vi "SWERVE_MODULE_ACT.vi"(4 "Steering Vel FF Kn":dbl=1.0 format="%#_13g", 5 "Drive Motor Info":T2={"Motor Name"="LF Drive", "MC type"=enum."Talon FX, P5", "Motor Type"=enum."NEO", "Gear Ratio"=0.0}, 6 "Drive Vel FF Kn":dbl=1.0 format="%#_13g", 7 "Steering Motor Info":T2={"Motor Name"="LF Steering", "MC type"=enum."Talon FX, P5", "Motor Type"=enum."NEO", "Gear Ratio"=0.0}, 8 "dt_Sec":dbl=0.02 format="%#_13g", 9 "Wheel Diameter IN":dbl=4.0 format="%#_13g", 10 "Swerve State":T3={"Speed"=0.0, "Angle"={"VALUE"=0.0, "COS"=1.0, "SIN"=0.0}} {"Angle"."SIN" format="%13.4f"; "Angle"."COS" format="%13.4f"; "Angle"."VALUE" format="%13.4f"}, 11 "Swerve Dmd":T3={"Speed"=0.0, "Angle"={"VALUE"=0.0, "COS"=1.0, "SIN"=0.0}} {"Angle"."SIN" format="%13.4f"; "Angle"."COS" format="%13.4f"; "Angle"."VALUE" format="%13.4f"}) -> ()   [LabVIEW 2023]
doc: "Creates a new SwerveModuleAct for an individual module with the specified swerve module state demand. \n\nParameters\n - Drive Vel FF Kn -- The normalization constant for Velocity FF on the Drive Motor.\n - Steering Vel FF Kn -- The normalization constant for Velocity FF on the Steering Motor."
uses:
  <vilib>/Rock Robotics/WPI/ThirdParty/JAS_Junk/TrajLib/TypeDef/SWERVE_DRIVE_MODULE_STATE.ctl
  <vilib>/Rock Robotics/WPI/ThirdParty/JAS_Junk/TrajLib/TypeDef/ROTATION2D.ctl
  <vilib>/Rock Robotics/WPI/ThirdParty/JAS_Junk/TrajLib/Enum/DCMOTOR_TYPES_ENUM.ctl
  <vilib>/Rock Robotics/WPI/ThirdParty/JAS_Junk/TrajLib/TypeDef/DCMOTOR_SIM.ctl
  <vilib>/Rock Robotics/WPI/ThirdParty/JAS_Junk/TrajLib/TypeDef/LINEAR_SYSTEM_SIM.ctl
  <vilib>/Rock Robotics/WPI/ThirdParty/JAS_Junk/TrajLib/TypeDef/LINEAR_SYSTEM.ctl
  <vilib>/Analysis/Matrix/Datatypes/RealMatrix.ctl
  <vilib>/Rock Robotics/WPI/ThirdParty/JAS_Junk/TrajLib/TypeDef/DCMOTOR.CTL
  <vilib>/Rock Robotics/WPI/ThirdParty/JAS_Junk/TrajLib/MathUtil_InputModulus.vi
  <vilib>/Rock Robotics/WPI/ThirdParty/JAS_Junk/TrajLib/DCMotor_GetCIM.vi
  <vilib>/Rock Robotics/WPI/ThirdParty/JAS_Junk/TrajLib/DCMotor_GetAndymark9015.vi
  <vilib>/Rock Robotics/WPI/ThirdParty/JAS_Junk/TrajLib/DCMotor_GetAndymarkRs775_125.vi
  <vilib>/Rock Robotics/WPI/ThirdParty/JAS_Junk/TrajLib/DCMotor_GetBag.vi
  <vilib>/Rock Robotics/WPI/ThirdParty/JAS_Junk/TrajLib/DCMotor_GetBanebotsRs550.vi
  <vilib>/Rock Robotics/WPI/ThirdParty/JAS_Junk/TrajLib/DCMotor_GetBanebotsRs775.vi
  <vilib>/Rock Robotics/WPI/ThirdParty/JAS_Junk/TrajLib/DCMotor_GetFalcon500.vi
  <vilib>/Rock Robotics/WPI/ThirdParty/JAS_Junk/TrajLib/DCMotor_GetMiniCIM.vi
  <vilib>/Rock Robotics/WPI/ThirdParty/JAS_Junk/TrajLib/DCMotor_GetNEO.vi
  <vilib>/Rock Robotics/WPI/ThirdParty/JAS_Junk/TrajLib/DCMotor_GetNEO550.vi
  <vilib>/Rock Robotics/WPI/ThirdParty/JAS_Junk/TrajLib/DCMotor_GetRomiBuiltIn.vi
  <vilib>/Rock Robotics/WPI/ThirdParty/JAS_Junk/TrajLib/DCMotor_GetVex775Pro.vi
  <vilib>/Rock Robotics/WPI/ThirdParty/JAS_Junk/TrajLib/VI/DCMotor_GetAndymarkAM2235A.vi
  <vilib>/Rock Robotics/WPI/ThirdParty/JAS_Junk/TrajLib/VI/DCMotor_GetAndymarkAM3493.vi
  <vilib>/Rock Robotics/WPI/ThirdParty/JAS_Junk/TrajLib/VI/DCMotor_GetFalcon500_FOC.vi
  <vilib>/Rock Robotics/WPI/ThirdParty/JAS_Junk/TrajLib/VI/DCMotor_GetKrakenX60.vi
  <vilib>/Rock Robotics/WPI/ThirdParty/JAS_Junk/TrajLib/VI/DCMotor_GetKrakenX60_FOC.vi
  <vilib>/Rock Robotics/WPI/ThirdParty/JAS_Junk/TrajLib/VI/DCMotor_GetNEOVortex.vi
  <vilib>/Rock Robotics/WPI/ThirdParty/JAS_Junk/TrajLib/Conv_Inches_Meters.vi
  <vilib>/Rock Robotics/WPI/ThirdParty/JAS_Junk/TrajLib/ProfiledPIDController_SetPID.vi
  <vilib>/Rock Robotics/WPI/ThirdParty/JAS_Junk/TrajLib/ProfiledPIDController_SetIntegratorRange.vi
  <vilib>/Rock Robotics/WPI/ThirdParty/JAS_Junk/TrajLib/ProfiledPIDController_SetTolerance_PosVel.vi
  <vilib>/Rock Robotics/WPI/ThirdParty/JAS_Junk/TrajLib/ProfiledPIDController_DisableContInput.vi
  <vilib>/Rock Robotics/WPI/ThirdParty/JAS_Junk/TrajLib/ProfiledPIDController_EnableContInput.vi
  <vilib>/Rock Robotics/WPI/ThirdParty/JAS_Junk/TrajLib/ProfiledPIDController_Reset_PosOnly.vi
  <vilib>/Rock Robotics/WPI/ThirdParty/JAS_Junk/TrajLib/ProfiledPIDController_NewPeriod.vi
  <vilib>/Rock Robotics/WPI/ThirdParty/JAS_Junk/TrajLib/ProfiledPIDController_Calculate_Meas_Goal.vi
  <vilib>/Rock Robotics/WPI/ThirdParty/JAS_Junk/TrajLib/ProfiledPIDController_AtGoal.vi
  <vilib>/Rock Robotics/WPI/ThirdParty/JAS_Junk/TrajLib/ProfiledPIDController_AtSetpoint.vi
  <vilib>/Rock Robotics/WPI/ThirdParty/JAS_Junk/TrajLib/ProfiledPIDController_SetConstraints.vi
  <vilib>/Rock Robotics/WPI/ThirdParty/JAS_Junk/TrajLib/SimpleMotorFF_Calculate.vi
  <vilib>/Rock Robotics/WPI/ThirdParty/JAS_Junk/TrajLib/PIDController_AtSetpoint.vi
  <vilib>/Rock Robotics/WPI/ThirdParty/JAS_Junk/TrajLib/PIDController_SetPIDF.vi
  <vilib>/Rock Robotics/WPI/ThirdParty/JAS_Junk/TrajLib/PIDController_SetDerivativeFilter.vi
  <vilib>/Rock Robotics/WPI/ThirdParty/JAS_Junk/TrajLib/PIDController_SetIntegratorRange.vi
  <vilib>/Rock Robotics/WPI/ThirdParty/JAS_Junk/TrajLib/PIDController_SetTolerancePandV.vi
  <vilib>/Rock Robotics/WPI/ThirdParty/JAS_Junk/TrajLib/PIDController_DisableContinousInput.vi
  <vilib>/Rock Robotics/WPI/ThirdParty/JAS_Junk/TrajLib/PIDController_EnableContinousInput.vi
  <vilib>/Rock Robotics/WPI/ThirdParty/JAS_Junk/TrajLib/PIDController_Reset.vi
  <vilib>/Rock Robotics/WPI/ThirdParty/JAS_Junk/TrajLib/PIDController_New.vi
  <vilib>/Rock Robotics/WPI/ThirdParty/JAS_Junk/TrajLib/PIDController_SetOutputLimits.vi
  <vilib>/Rock Robotics/WPI/ThirdParty/JAS_Junk/TrajLib/VI/PIDController_SetIntegratorZone.vi
  <vilib>/Rock Robotics/WPI/ThirdParty/JAS_Junk/TrajLib/DCMotor_New.vi
  <vilib>/Rock Robotics/WPI/ThirdParty/JAS_Junk/TrajLib/PIDController_SetPID.vi
  <vilib>/Rock Robotics/WPI/ThirdParty/JAS_Junk/TrajLib/TrapProfState_New.vi
  <vilib>/Rock Robotics/WPI/ThirdParty/JAS_Junk/TrajLib/ProfiledPIDController_Reset.vi
  <vilib>/Rock Robotics/WPI/ThirdParty/JAS_Junk/TrajLib/PIDController_NewPeriod.vi
  <vilib>/Rock Robotics/SystemInterfaces/NetworkCommunication/NetComm_UsageReport_report.vi
  <vilib>/Rock Robotics/WPI/ThirdParty/JAS_Junk/TrajLib/ProfiledPIDController_SetGoal_PosOnly.vi
  <vilib>/Rock Robotics/WPI/ThirdParty/JAS_Junk/TrajLib/ProfiledPIDController_Calculate_Meas.vi
  <vilib>/Rock Robotics/WPI/ThirdParty/JAS_Junk/TrajLib/TrapProfState_Equals.vi
  <vilib>/Rock Robotics/WPI/ThirdParty/JAS_Junk/TrajLib/ProfiledPIDController_SetGoal.vi
  <vilib>/Rock Robotics/WPI/ThirdParty/JAS_Junk/TrajLib/PIDController_Calculate_SP_PV.vi
  <vilib>/Rock Robotics/WPI/ThirdParty/JAS_Junk/TrajLib/TrapProfile_New.vi
  <vilib>/Rock Robotics/WPI/ThirdParty/JAS_Junk/TrajLib/ProfiledPIDController_GetPeriod.vi
  <vilib>/Rock Robotics/WPI/ThirdParty/JAS_Junk/TrajLib/TrapProfile_Calculate.vi
  <vilib>/Rock Robotics/WPI/ThirdParty/JAS_Junk/TrajLib/ControllerUtil_GetModulusError.vi
  <vilib>/Rock Robotics/WPI/ThirdParty/JAS_Junk/TrajLib/PIDController_SetSetpoint.vi
  <vilib>/Rock Robotics/WPI/ThirdParty/JAS_Junk/TrajLib/PIDController_Calculate_PV.vi
  <vilib>/Rock Robotics/WPI/ThirdParty/JAS_Junk/TrajLib/TrapProfile_ShouldFlipAcceleration.vi
  <vilib>/Rock Robotics/WPI/ThirdParty/JAS_Junk/TrajLib/TrapProfile_Direct.vi
  <vilib>/Rock Robotics/WPI/ThirdParty/JAS_Junk/TrajLib/PIDController_GetPeriod.vi
  <vilib>/Rock Robotics/Network Tables/NT Read Variant.vi
  <vilib>/Rock Robotics/WPI/ThirdParty/JAS_Junk/TrajLib/Globals/Util_LibraryGlobals.vi
  <vilib>/Rock Robotics/Network Tables/NT Write Variant.vi
  <vilib>/Rock Robotics/WPI/ThirdParty/JAS_Junk/TrajLib/PIDController_AdvCalculate_FF_Sp_Pv.vi
  <vilib>/Rock Robotics/WPI/ThirdParty/Phoenix-LabVIEW/Motor Controller/Controls/CTRE_Phoenix_MotorControl_ControlMode.ctl
  <vilib>/Rock Robotics/WPI/ThirdParty/JAS_Junk/TrajLib/Trajectory_Library.lvlib
  <vilib>/Rock Robotics/WPI/ThirdParty/REV Robotics/REVLib/Typedef/Spark MAX Control Type.ctl
  <vilib>/Analysis/Matrix/NI_Matrix.lvlib
  <vilib>/Rock Robotics/WPI/ThirdParty/Phoenix6/controls/VelocityDutyCycle SetControl.vi
  <vilib>/Rock Robotics/WPI/ThirdParty/Phoenix6/getters/GetPRO_PosAndVel_Position.vi
  <vilib>/Rock Robotics/WPI/ThirdParty/Phoenix6/controls/PositionDutyCycle SetControl.vi
  <vilib>/Rock Robotics/WPI/ThirdParty/Phoenix6/getters/GetPRO_PosAndVel_Velocity.vi
  <vilib>/Rock Robotics/WPI/ThirdParty/Phoenix-LabVIEW/Motor Controller/Get/CTRE_Phoenix_MotorController_GetSelectedSensorData.vi
  <vilib>/Rock Robotics/WPI/ThirdParty/REV Robotics/REVLib/SubVI/Public/SPARK Get Encoder Status Position.vi
  <vilib>/Rock Robotics/WPI/ThirdParty/REV Robotics/REVLib/SubVI/Public/SPARK Get Encoder Status Velocity.vi
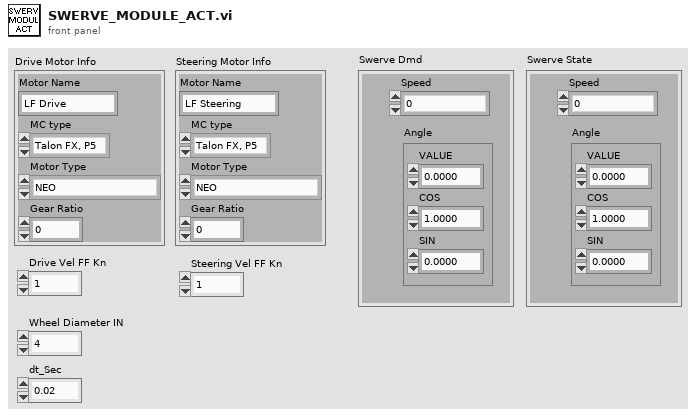
[diagram p1: front panel]
types:
  T1 = typedef "Trajectory_Library.lvlib/DCMOTOR_TYPES_ENUM.ctl" = enum16{"CIM", "AndyMark 9015", "Andy Mark RS 775 125", "Bag", "BaneBots RS 550", "BaneBots RS 775", "Falcon 500", "Mini CIM", "NEO", "NEO 550", "Romi BuiltIn", "Vex 775 Pro", "Snow Blower AM 2235A", "Bosch Seat AM 3493", "Falcon 500 FOC", "Kraken X60", "Kraken X60 FOC", "NEO Vortex"}
  T2 = cluster{"Motor Name":string, "MC type":enum16{"Talon FX, P5", "Talon FX, P6", "SPARK MAX"}, "Motor Type":T1, "Gear Ratio":dbl}
  T3 = typedef "Trajectory_Library.lvlib/SWERVE_DRIVE_MODULE_STATE.ctl" = cluster{"Speed":dbl, "Angle":T4}
  T4 = typedef "Trajectory_Library.lvlib/ROTATION2D.ctl" = cluster{"VALUE":dbl, "COS":dbl, "SIN":dbl}
  T5 = enum16{"Talon FX, P5", "Talon FX, P6", "SPARK MAX"}
  T6 = enum16{"DemandType_Neutral", "DemandType_AuxPID", "DemandType_ArbitraryFeedForward"}
  T7 = typedef "Spark MAX Control Type.ctl" = enum16{"Percent VBus", "Voltage", "Velocity", "Position", "Smart Motion", "Current", "Smart Velocity", "MAXMotion Position", "MAXMotion Velocity"}
  T8 = cluster{"Future Proof Configs":bool, "MotorOutputInverted":u16, "MotorOutputNeutralMode":u16, "MotorOutputDutyCycleNeutralDeadband":dbl, "MotorOutputPeakForwardDutyCycle":dbl, "MotorOutputPeakReverseDutyCycle":dbl, "MotorOutputControlTimesyncFreqHz":dbl, "CurrentLimitsStatorCurrentLimit":dbl, "CurrentLimitsStatorCurrentLimitEnable":bool, "CurrentLimitsSupplyCurrentLimit":dbl, "CurrentLimitsSupplyCurrentLimitEnable":bool, "CurrentLimitsSupplyCurrentLowerLimit":dbl, "CurrentLimitsSupplyCurrentLowerTime":dbl, "VoltageSupplyVoltageTimeConstant":dbl, "VoltagePeakForwardVoltage":dbl, "VoltagePeakReverseVoltage":dbl, "TorqueCurrentPeakForwardTorqueCurrent":dbl, "TorqueCurrentPeakReverseTorqueCurrent":dbl, "TorqueCurrentTorqueNeutralDeadband":dbl, "FeedbackFeedbackRotorOffset":dbl, "FeedbackSensorToMechanismRatio":dbl, "FeedbackRotorToSensorRatio":dbl, "FeedbackFeedbackSensorSource":u16, "FeedbackFeedbackRemoteSensorID":i16, "FeedbackVelocityFilterTimeConstant":dbl, "DifferentialSensorsDifferentialSensorSource":u16, "DifferentialSensorsDifferentialTalonFXSensorID":i16, "DifferentialSensorsDifferentialRemoteSensorID":i16, "DifferentialConstantsPeakDifferentialDutyCycle":dbl, "DifferentialConstantsPeakDifferentialVoltage":dbl, "DifferentialConstantsPeakDifferentialTorqueCurrent":dbl, "OpenLoopRampsDutyCycleOpenLoopRampPeriod":dbl, "OpenLoopRampsVoltageOpenLoopRampPeriod":dbl, "OpenLoopRampsTorqueOpenLoopRampPeriod":dbl, "ClosedLoopRampsDutyCycleClosedLoopRampPeriod":dbl, "ClosedLoopRampsVoltageClosedLoopRampPeriod":dbl, "ClosedLoopRampsTorqueClosedLoopRampPeriod":dbl, "HardwareLimitSwitchForwardLimitType":u16, "HardwareLimitSwitchForwardLimitAutosetPositionEnable":bool, "HardwareLimitSwitchForwardLimitAutosetPositionValue":dbl, "HardwareLimitSwitchForwardLimitEnable":bool, "HardwareLimitSwitchForwardLimitSource":u16, "HardwareLimitSwitchForwardLimitRemoteSensorID":i16, "HardwareLimitSwitchReverseLimitType":u16, "HardwareLimitSwitchReverseLimitAutosetPositionEnable":bool, "HardwareLimitSwitchReverseLimitAutosetPositionValue":dbl, "HardwareLimitSwitchReverseLimitEnable":bool, "HardwareLimitSwitchReverseLimitSource":u16, "HardwareLimitSwitchReverseLimitRemoteSensorID":i16, "AudioBeepOnBoot":bool, "AudioBeepOnConfig":bool, "AudioAllowMusicDurDisable":bool, "SoftwareLimitSwitchForwardSoftLimitEnable":bool, "SoftwareLimitSwitchReverseSoftLimitEnable":bool, "SoftwareLimitSwitchForwardSoftLimitThreshold":dbl, "SoftwareLimitSwitchReverseSoftLimitThreshold":dbl, "MotionMagicMotionMagicCruiseVelocity":dbl, "MotionMagicMotionMagicAcceleration":dbl, "MotionMagicMotionMagicJerk":dbl, "MotionMagicMotionMagicExpo_kV":dbl, "MotionMagicMotionMagicExpo_kA":dbl, "CustomParamsCustomParam0":i16, "CustomParamsCustomParam1":i16, "ClosedLoopGeneralContinuousWrap":bool, "Slot0kP":dbl, "Slot0kI":dbl, "Slot0kD":dbl, "Slot0kS":dbl, "Slot0kV":dbl, "Slot0kA":dbl, "Slot0kG":dbl, "Slot0GravityType":u16, "Slot0StaticFeedforwardSign":u16, "Slot1kP":dbl, "Slot1kI":dbl, "Slot1kD":dbl, "Slot1kS":dbl, "Slot1kV":dbl, "Slot1kA":dbl, "Slot1kG":dbl, "Slot1GravityType":u16, "Slot1StaticFeedforwardSign":u16, "Slot2kP":dbl, "Slot2kI":dbl, "Slot2kD":dbl, "Slot2kS":dbl, "Slot2kV":dbl, "Slot2kA":dbl, "Slot2kG":dbl, "Slot2GravityType":u16, "Slot2StaticFeedforwardSign":u16}
  T9 = typedef "Trajectory_Library.lvlib/DCMOTOR_SIM.ctl" = cluster{"LinearSystemSim":T10, "GearBox":T13, "Gearing":dbl}
  T10 = typedef "Trajectory_Library.lvlib/LINEAR_SYSTEM_SIM.ctl" = cluster{"m_Plant":T11, "m_X":T12, "m_Y":T12, "m_U":T12, "MeasureStdDev":T12}
  T11 = typedef "Trajectory_Library.lvlib/LINEAR_SYSTEM.ctl" = cluster{"m_A":T12, "m_B":T12, "m_C":T12, "m_D":T12, "States":i32, "Inputs":i32, "Outputs":i32}
  T12 = typedef "NI_Matrix.lvlib/RealMatrix.ctl" = dbl[][]
  T13 = typedef "Trajectory_Library.lvlib/DCMOTOR.CTL" = cluster{"nominalVoltage_Volts":dbl, "StallTorque_NM":dbl, "StallCurrent_Amps":dbl, "FreeCurrent_Amps":dbl, "FreeSpeed_RadPerSec":dbl, "R_Ohms":dbl, "KvINV_RadPerSecPerVolt":dbl, "Kt_NMPerAmp":dbl, "L_H":dbl, "Jr_KgM2":dbl}
  T14 = typedef "CTRE_Phoenix_MotorControl_ControlMode.ctl" = u16
  T15 = typedef "Trajectory_Library.lvlib/SIMPLE_MOTOR_FF.ctl" = cluster{"Ks":dbl, "Kv":dbl, "Ka":dbl, "KnInv":dbl}
  T16 = typedef "WPI_MotorControlDeviceRef.ctl" = cluster{"DeviceStatus":errorcluster, "Type":T17, "PWM":cluster{"PWM Channel":T18, "DeadBand":T19}, "CAN":cluster{"Device Number":u8, "SetOutput VI Ref":variant, "GetOutput VI Ref":variant, "Enable VI Ref":variant, "Disable VI Ref":variant, "Data":variant}, "Invert":bool, "DIO PWM":cluster{"PWM \"Enable\" Channel":T18, "DIOChannel":T20, "PWM Rate":dbl}}
  T17 = typedef "WPI_MotorControlType.ctl" = enum16{"PWM", "CAN", "DIO PWM"}
  T18 = typedef "FPGA_DIOPWMChannel.ctl" = enum8{"PWM 0", "PWM 1", "PWM 2", "PWM 3", "PWM 4", "PWM 5", "PWM 6", "PWM 7", "PWM 8", "PWM 9", "PWM MXP 0", "PWM MXP 1", "PWM MXP 2", "PWM MXP 3", "PWM MXP 4", "PWM MXP 5", "PWM MXP 6", "PWM MXP 7", "PWM MXP 8", "PWM MXP 9", "Invalid"}
  T19 = typedef "WPI_PWMDeadband.ctl" = cluster{"Name":string, "maxPositivePwm":i32, "minPositivePwm":i32, "centerPwm":i32, "maxNegativePwm":i32, "minNegativePwm":i32, "angularRange":u16}
  T20 = typedef "FPGA_DIOChannel.ctl" = enum8{"DIO 0", "DIO 1", "DIO 2", "DIO 3", "DIO 4", "DIO 5", "DIO 6", "DIO 7", "DIO 8", "DIO 9", "DIO MXP 0", "DIO MXP 1", "DIO MXP 2", "DIO MXP 3", "DIO MXP 4", "DIO MXP 5", "DIO MXP 6", "DIO MXP 7", "DIO MXP 8", "DIO MXP 9", "DIO MXP 10", "DIO MXP 11", "DIO MXP 12", "DIO MXP 13", "DIO MXP 14", "DIO MXP 15", "SPI Port CS1", "SPI Port CS2", "SPI Port CS3", "SPI Port MISO", "SPI Port MOSI", "Invalid"}
  T21 = typedef "DeviceReference.ctl" = cluster{"CANbus Name":string, "Device Encoding":u32, "Device Name":string}
  T22 = cluster{"Value":dbl, "System Timestamp":dbl, "CANivore Timestamp":dbl, "ECU Timestamp":dbl}
  T23 = typedef "Trajectory_Library.lvlib/PID_ADV_TUNING.ctl" = cluster{"Kf":dbl, "Kp":dbl, "Ki":dbl, "Kd":dbl, "MaximumIntegral":dbl, "MinimumIntegral":dbl, "Filter Derivative":bool, "IntegralZone":dbl}
  T24 = typedef "Trajectory_Library.lvlib/TRAPEZOID_PROFILE_CONSTRAINT.ctl" = cluster{"MaxVelocity":dbl, "MaxAcceleration":dbl}
  T25 = typedef "Trajectory_Library.lvlib/PID_INPUT_LIMITS.ctl" = cluster{"MaxInput":dbl, "MinInput":dbl, "Continuous":bool}
  T26 = typedef "Trajectory_Library.lvlib/PID_TUNING.ctl" = cluster{"Kp":dbl, "Ki":dbl, "Kd":dbl, "MaximumIntegral":dbl, "MinimumIntegral":dbl, "IntegralZone":dbl}
  T27 = typedef "Trajectory_Library.lvlib/PID_ADV_LIMITS.ctl" = cluster{"MaxInput":dbl, "MinInput":dbl, "Continuous":bool, "MaxOutput":dbl, "MinOutput":dbl}
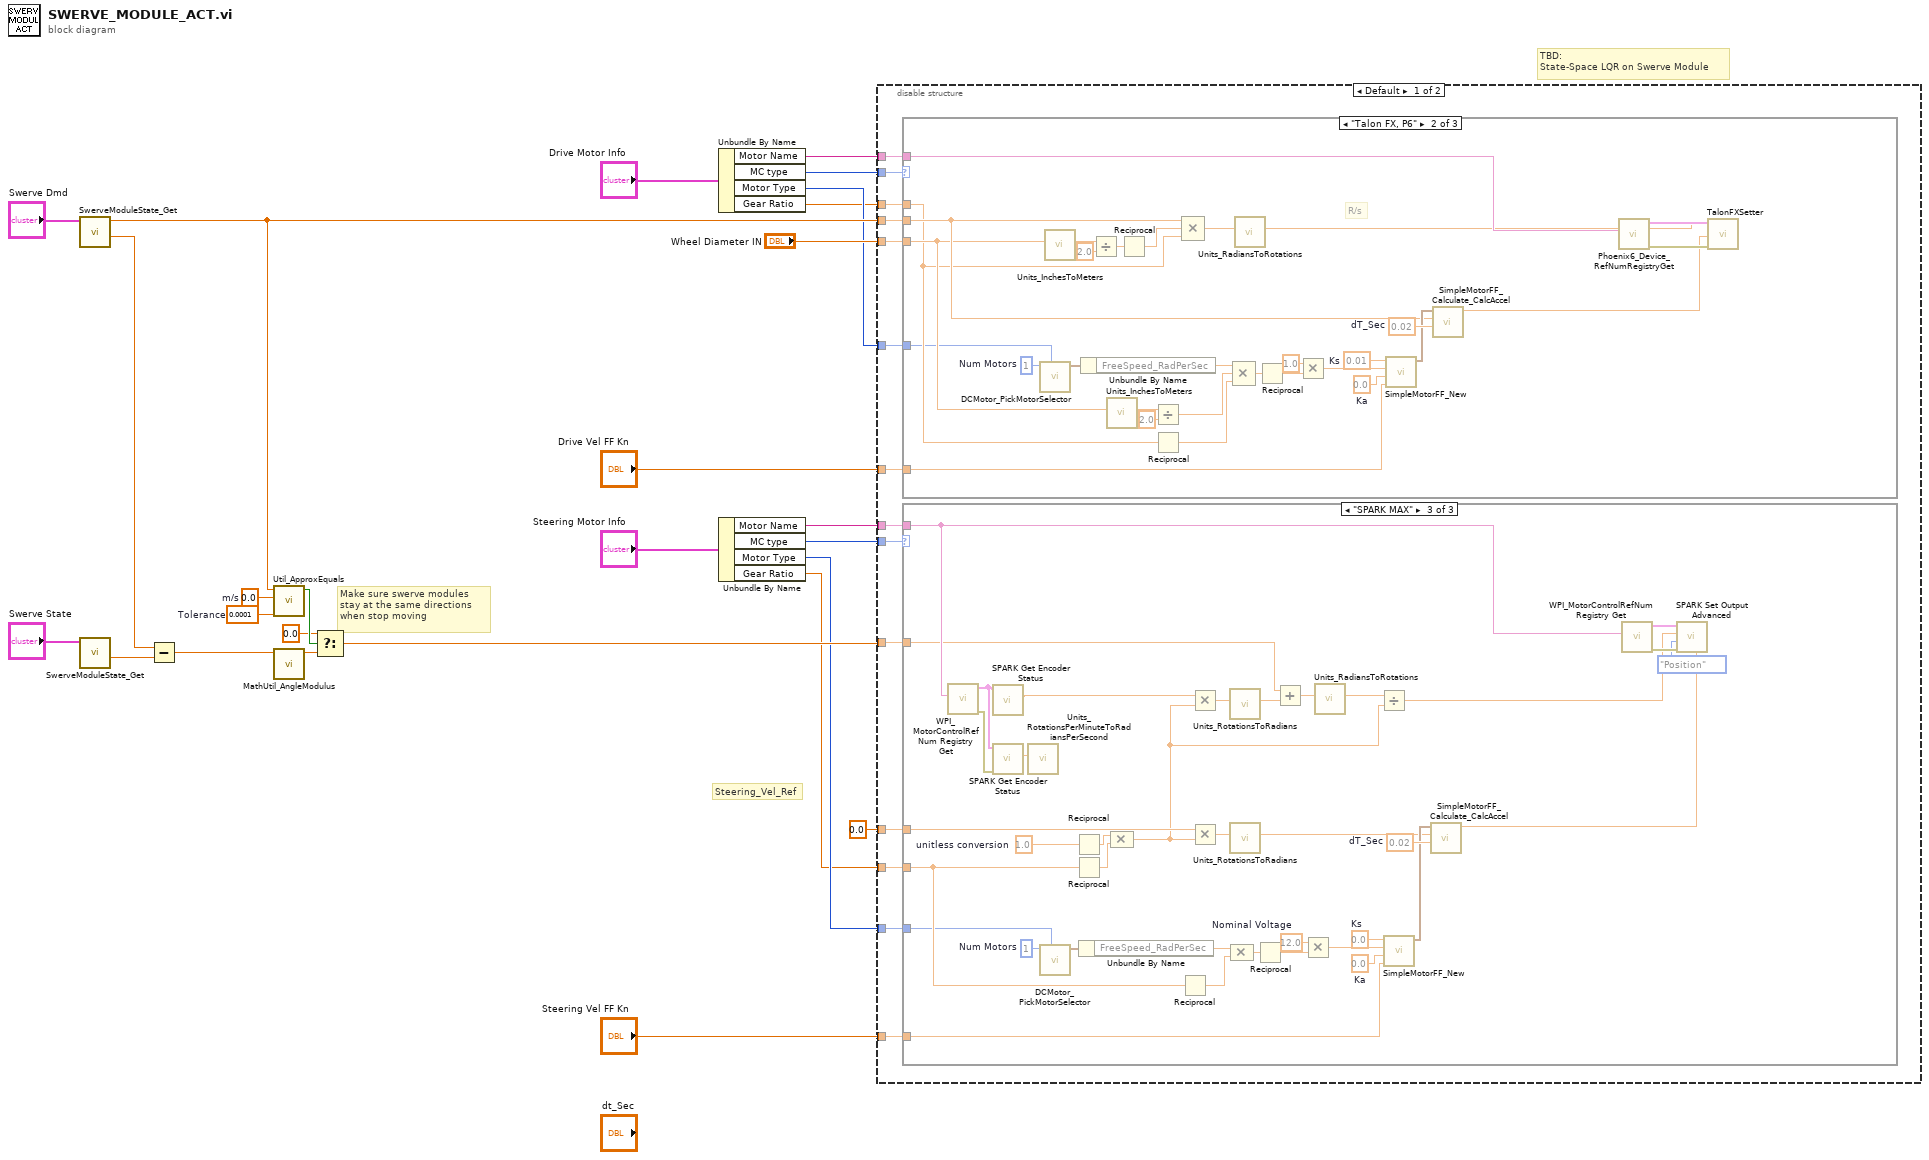
[diagram p0: block diagram]
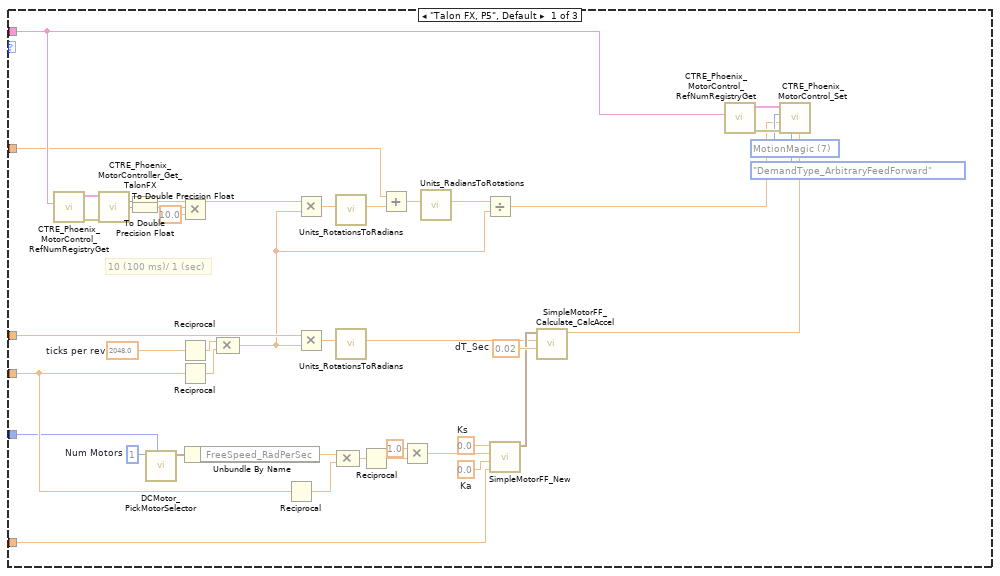
[diagram p2: hidden frame]
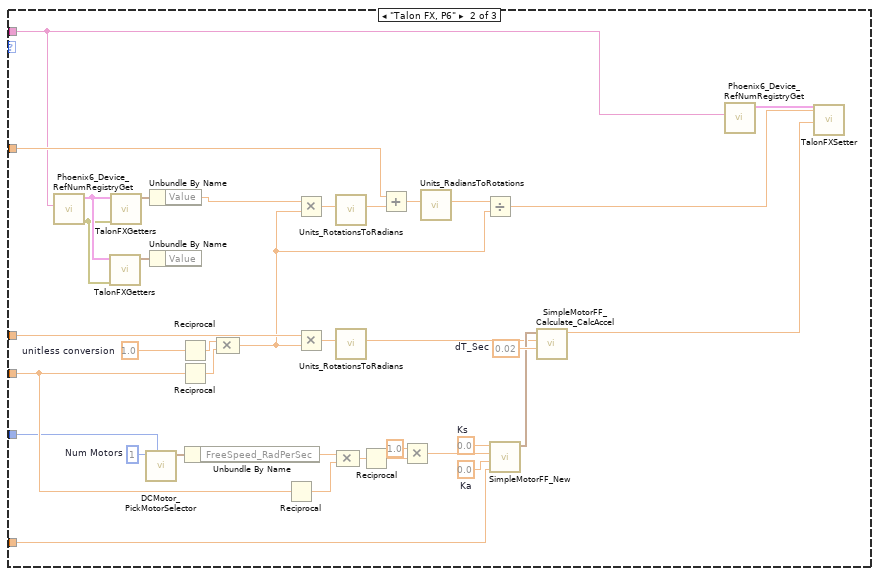
[diagram p3: hidden frame]
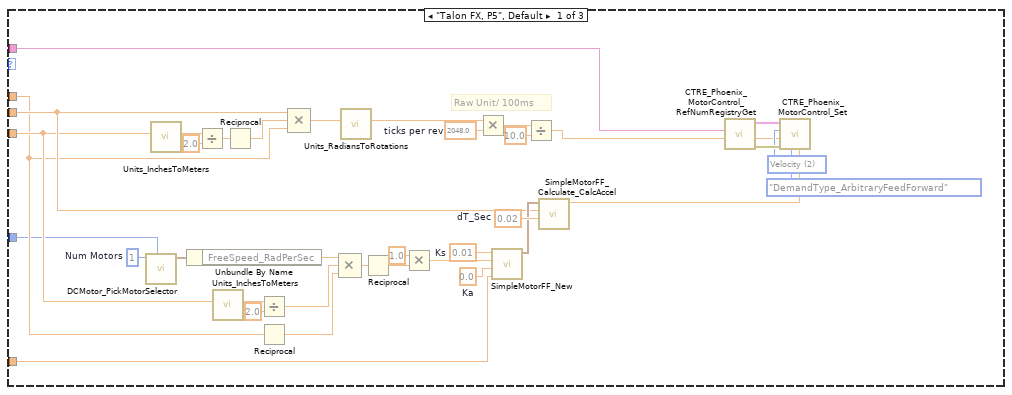
[diagram p4: hidden frame]
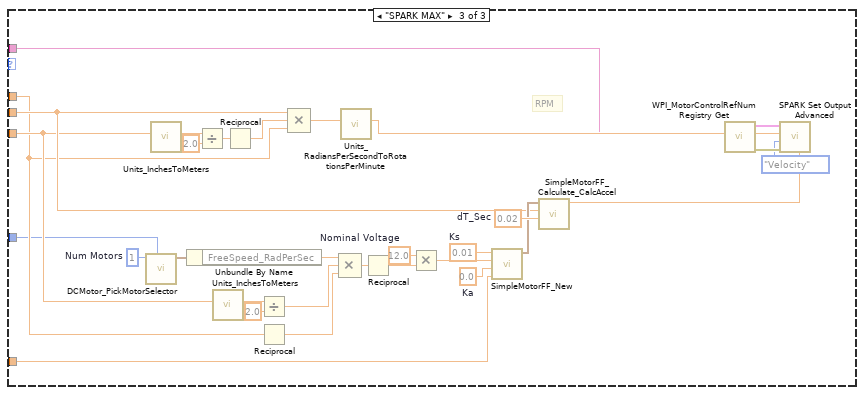
[diagram p5: hidden frame]
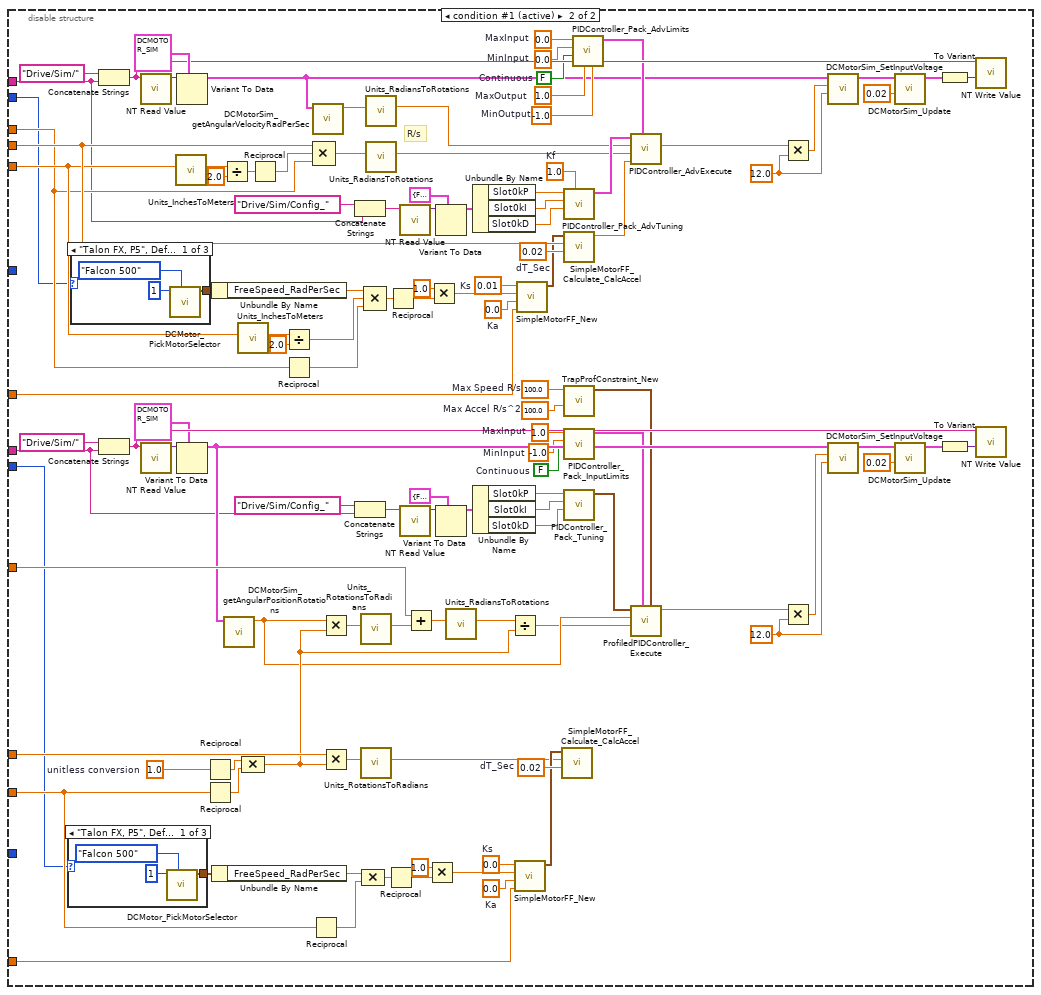
[diagram p6: hidden frame]
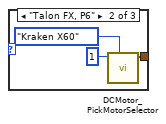
[diagram p7: hidden frame]
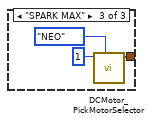
[diagram p8: hidden frame]
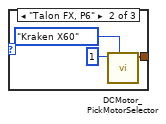
[diagram p9: hidden frame]
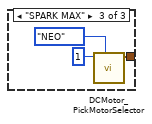
[diagram p10: hidden frame]
diagram:
  w22 = 0.0001  # Tolerance
  w23 = 0.0  # m/s
  # "Steering_Vel_Ref"
  # "TBD:\nState-Space LQR on Swerve Module"
  # "Make sure swerve modules \nstay at the same directions \nwhen stop moving"
  n1 = call <vilib>:"SwerveModuleState_Get.vi"("Desired State"="Swerve Dmd") -> ("Angle RADIANS"=w19:dbl, "Speed M/S"=w20:dbl)  [unwired: 9 in]
  n2 = call <vilib>:"SwerveModuleState_Get.vi"("Desired State"="Swerve State") -> ("Angle RADIANS"=w18:dbl)  [unwired: 9 in, 1 out]
  n3 = Subtract(x=w19, y=w18) -> (x-y=w1:dbl)
  n4 = call <vilib>:"Util_ApproxEquals.vi"("Tolerance"=w22, "Value 2"=w23, "Value 1"=w20) -> ("ApproxEquals"=w21:bool)  [unwired: 8 in]
  n5 = call <vilib>:"MathUtil_AngleModulus.vi"("InputAngle"=w1) -> ("ModulsAngle"=w2:dbl)  [unwired: 10 in]
  n6 = Select(t=0.0, s=w21, f=w2) -> (s? t:f=w17:dbl)
  n7 = Unbundle By Name("Drive Motor Info") -> ("Motor Name"=w6:string, "MC type"=w9:T5, "Motor Type"=w10:T1, "Gear Ratio"=w7:dbl)
  n8 = Unbundle By Name("Steering Motor Info") -> ("Motor Name"=w5:string, "MC type"=w13:T5, "Motor Type"=w12:T1, "Gear Ratio"=w8:dbl)
  n9 = disable-structure shown="Default" {
    disable-tunnel: 0.0 ("Radians") -> [w40 w365]
    disable-tunnel: w20 -> [w39 w364]
    disable-tunnel: w17 -> [w38 w363]
    disable-tunnel: "Wheel Diameter IN" -> [w37 w362]
    disable-tunnel: w13 -> [w36 w256]
    disable-tunnel: w12 -> [w35 _]
    disable-tunnel: w10 -> [w34 _]
    disable-tunnel: w9 -> [w33 w254]
    disable-tunnel: w8 -> [w32 w361]
    disable-tunnel: w7 -> [w31 w360]
    disable-tunnel: w6 -> [w30 w276]
    disable-tunnel: w5 -> [w29 w295]
    disable-tunnel: "Steering Vel FF Kn" -> [w28 w359]
    disable-tunnel: "Drive Vel FF Kn" -> [w27 w358]
    frame condition #0 {
      n10 = case shown="\"Talon FX, P6\"" w33 {
        tunnel: w39 -> [w166 w202 w228]
        tunnel: w30 -> [w165 w196 w226]
        tunnel: w31 -> [w162 w200 w225]
        tunnel: w34 -> [w155 w194 w221]
        tunnel: w37 -> [w163 w201 w227]
        tunnel: w27 -> [w158 w199 w224]
        frame "Talon FX, P5", Default {
          w176 = 2048.0  # ticks per rev
          w156 = 1  # Num Motors
          w173 = 0.02  # dT_Sec
          w184 = 0.01  # Ks
          w183 = 0.0  # Ka
          w175 = T14 2 items=["PercentOutput"=0, "Position"=1, "Velocity"=2, "Current"=3, "Follower"=5, "MotionProfile"=6, "MotionMagic"=7, "MotionProfileArc"=10, "Disabled"=15] ("Control Mode")
          # "Raw Unit/ 100ms"
          n11 = call <vilib>:"DCMotor_PickMotorSelector.vi"("DCMOTOR_TYPES"=w155, "Num Motors"=w156) -> ("DCMOTOR"=w157:T13)  [unwired: 9 in]
          n12 = call <vilib>:"Units_InchesToMeters.vi"("Inches"=w163) -> ("Meters"=w187:dbl)  [unwired: 10 in]
          n13 = Unbundle By Name(w157) -> ("FreeSpeed_RadPerSec"=w178:dbl)
          n14 = Divide(x=w187, y=2.0) -> (x/y=w186:dbl)
          n15 = call <vilib>:"Units_InchesToMeters.vi"("Inches"=w163) -> ("Meters"=w182:dbl)  [unwired: 10 in]
          n16 = Reciprocal(x=w186) -> (1/x=w185:dbl)
          n17 = Divide(x=w182, y=2.0) -> (x/y=w180:dbl)
          n18 = Reciprocal(x=w162) -> (1/x=w179:dbl)
          n19 = Compound Arithmetic op=MULTIPLY(w166, w185, w162) -> (w171:dbl)
          n20 = Compound Arithmetic op=MULTIPLY(w178, w180, w179) -> (w177:dbl)
          n21 = call <vilib>:"Units_RadiansToRotations.vi"("Radians"=w171) -> ("Rotations"=w170:dbl)  [unwired: 10 in]
          n22 = Reciprocal(x=w177) -> (1/x=w168:dbl)
          n23 = Multiply(x=1.0, y=w168) -> (x*y=w167:dbl)
          n24 = Multiply(x=w170, y=w176) -> (x*y=w160:dbl)
          n25 = call <vilib>:"SimpleMotorFF_New.vi"("Kn"=w158, "Ka"=w183, "Kv"=w167, "Ks"=w184) -> ("SIMPLE_MOTOR_FF"=w172:T15)  [unwired: 7 in]
          n26 = Divide(x=w160, y=10.0) -> (x/y=w159:dbl)
          n27 = call <vilib>:"SimpleMotorFF_Calculate_CalcAccel.vi"("dT_Sec"=w173, "VelSp"=w166, "SIMPLE_MOTOR_FF"=w172) -> ("FeedForward"=w164:dbl)  [unwired: 8 in]
          n28 = call <vilib>:"CTRE_Phoenix_MotorControl_RefNumRegistryGet.vi"("refnum name"=w165) -> ("error out"=w189:errorcluster, "PhoenixMotorControlDevRef"=w190:T16)  [unwired: 9 in]
          n29 = call <vilib>:"CTRE_Phoenix_MotorControl_Set.vi"("Demand1"=w164, "DemandType"=T6."DemandType_ArbitraryFeedForward", "error in (no error)"=w189, "Output"=w159, "Control Mode"=w175, "PhoenixMotorControlDevRef"=w190) -> ()  [unwired: 4 in, 2 out]
        }
        frame "Talon FX, P6" {
          w193 = 1  # Num Motors
          w208 = 0.02  # dT_Sec
          w216 = 0.01  # Ks
          w215 = 0.0  # Ka
          # "R/s"
          n30 = call <vilib>:"DCMotor_PickMotorSelector.vi"("DCMOTOR_TYPES"=w194, "Num Motors"=w193) -> ("DCMOTOR"=w195:T13)  [unwired: 9 in]
          n31 = call <vilib>:"Units_InchesToMeters.vi"("Inches"=w201) -> ("Meters"=w219:dbl)  [unwired: 10 in]
          n32 = Unbundle By Name(w195) -> ("FreeSpeed_RadPerSec"=w210:dbl)
          n33 = Divide(x=w219, y=2.0) -> (x/y=w218:dbl)
          n34 = call <vilib>:"Units_InchesToMeters.vi"("Inches"=w201) -> ("Meters"=w214:dbl)  [unwired: 10 in]
          n35 = Reciprocal(x=w218) -> (1/x=w217:dbl)
          n36 = Divide(x=w214, y=2.0) -> (x/y=w212:dbl)
          n37 = Reciprocal(x=w200) -> (1/x=w211:dbl)
          n38 = Compound Arithmetic op=MULTIPLY(w202, w217, w200) -> (w206:dbl)
          n39 = Compound Arithmetic op=MULTIPLY(w210, w212, w211) -> (w209:dbl)
          n40 = call <vilib>:"Units_RadiansToRotations.vi"("Radians"=w206) -> ("Rotations"=w191:dbl)  [unwired: 10 in]
          n41 = Reciprocal(x=w209) -> (1/x=w204:dbl)
          n42 = Multiply(x=1.0, y=w204) -> (x*y=w203:dbl)
          n43 = call <vilib>:"SimpleMotorFF_New.vi"("Kn"=w199, "Ka"=w215, "Kv"=w203, "Ks"=w216) -> ("SIMPLE_MOTOR_FF"=w207:T15)  [unwired: 7 in]
          n44 = call <vilib>:"SimpleMotorFF_Calculate_CalcAccel.vi"("dT_Sec"=w208, "VelSp"=w202, "SIMPLE_MOTOR_FF"=w207) -> ("FeedForward"=w192:dbl)  [unwired: 8 in]
          n45 = call <vilib>:"Phoenix6_Device_RefNumRegistryGet.vi"("refnum name"=w196) -> ("error out"=w197:errorcluster, "data"=w198:T21)  [unwired: 9 in]
          n46 = call-poly <vilib>:"TalonFXSetter.vi"("DeviceReference"=w198, "Velocity"=w191, "FeedForward"=w192, "error in"=w197) -> ()  [unwired: 22 in, 2 out]
        }
        frame "SPARK MAX" {
          w234 = 12.0  # Nominal Voltage
          w222 = 1  # Num Motors
          w237 = 0.02  # dT_Sec
          w245 = 0.01  # Ks
          w244 = 0.0  # Ka
          # "RPM"
          n47 = call <vilib>:"DCMotor_PickMotorSelector.vi"("DCMOTOR_TYPES"=w221, "Num Motors"=w222) -> ("DCMOTOR"=w223:T13)  [unwired: 9 in]
          n48 = call <vilib>:"Units_InchesToMeters.vi"("Inches"=w227) -> ("Meters"=w248:dbl)  [unwired: 10 in]
          n49 = Unbundle By Name(w223) -> ("FreeSpeed_RadPerSec"=w239:dbl)
          n50 = Divide(x=w248, y=2.0) -> (x/y=w247:dbl)
          n51 = call <vilib>:"Units_InchesToMeters.vi"("Inches"=w227) -> ("Meters"=w243:dbl)  [unwired: 10 in]
          n52 = Reciprocal(x=w247) -> (1/x=w246:dbl)
          n53 = Divide(x=w243, y=2.0) -> (x/y=w241:dbl)
          n54 = Reciprocal(x=w225) -> (1/x=w240:dbl)
          n55 = Compound Arithmetic op=MULTIPLY(w228, w246, w225) -> (w235:dbl)
          n56 = Compound Arithmetic op=MULTIPLY(w239, w241, w240) -> (w238:dbl)
          n57 = call <vilib>:"Units_RadiansPerSecondToRotationsPerMinute.vi"("RadiansPerSecond"=w235) -> ("RotationsPerMinute"=w230:dbl)  [unwired: 10 in]
          n58 = Reciprocal(x=w238) -> (1/x=w233:dbl)
          n59 = Multiply(x=w234, y=w233) -> (x*y=w232:dbl)
          n60 = call <vilib>:"SimpleMotorFF_New.vi"("Kn"=w224, "Ka"=w244, "Kv"=w232, "Ks"=w245) -> ("SIMPLE_MOTOR_FF"=w236:T15)  [unwired: 7 in]
          n61 = call <vilib>:"SimpleMotorFF_Calculate_CalcAccel.vi"("dT_Sec"=w237, "VelSp"=w228, "SIMPLE_MOTOR_FF"=w236) -> ("FeedForward"=w229:dbl)  [unwired: 8 in]
          n62 = call <vilib>:"WPI_MotorControlRefNum Registry Get.vi"("refnum name"=w226) -> ("error out"=w250:errorcluster, "MotorControlDevRef"=w251:T16)  [unwired: 9 in]
          n63 = call <vilib>:"SPARK Set Output Advanced.vi"("Arbitrary Feed Forward (0)"=w229, "error in (no error)"=w250, "Control Mode"=Spark_MAX_Control_Type."Velocity", "Setpoint"=w230, "MotorControlDevRef"=w251) -> ()  [unwired: 5 in, 2 out]
        }
      }
      n64 = case shown="\"SPARK MAX\"" w36 {
        tunnel: w40 -> [w54 w102 w135]
        tunnel: w29 -> [w56 w89 w136]
        tunnel: w38 -> [w50 w99 w130]
        tunnel: w32 -> [w45 w95 w126]
        tunnel: w35 -> [w41 w82 w122]
        tunnel: w28 -> [w44 w94 w125]
        frame "Talon FX, P5", Default {
          w66 = 2048.0  # ticks per rev
          w70 = 0.02  # dT_Sec
          w42 = 1  # Num Motors
          w77 = 0.0  # Ks
          w76 = 0.0  # Ka
          w79 = T14 7 items=["PercentOutput"=0, "Position"=1, "Velocity"=2, "Current"=3, "Follower"=5, "MotionProfile"=6, "MotionMagic"=7, "MotionProfileArc"=10, "Disabled"=15] ("Control Mode")
          # "10 (100 ms)/ 1 (sec)"
          n65 = call <vilib>:"CTRE_Phoenix_MotorControl_RefNumRegistryGet.vi"("refnum name"=w56) -> ("error out"=w60:errorcluster, "PhoenixMotorControlDevRef"=w61:T16)  [unwired: 9 in]
          n66 = call-poly <vilib>:"CTRE_Phoenix_MotorController_Get_TalonFX.vi"("PhoenixMotorControlDevRef"=w61, "error in"=w60) -> ("Position (Raw Sensor Units)"=w62:i32, "Velocity (Raw Sensor Units per 100 ms)"=w59:i32)  [unwired: 10 in, 2 out]
          n67 = To Double Precision Float(number=w62) -> (double precision float=w53:dbl)
          n68 = To Double Precision Float(number=w59) -> (double precision float=w57:dbl)
          n69 = call <vilib>:"DCMotor_PickMotorSelector.vi"("DCMOTOR_TYPES"=w41, "Num Motors"=w42) -> ("DCMOTOR"=w43:T13)  [unwired: 9 in]
          n70 = Multiply(x=w57, y=10.0) -> ()  [unwired: 1 out]
          n71 = Reciprocal(x=w66) -> (1/x=w64:dbl)
          n72 = Reciprocal(x=w45) -> (1/x=w65:dbl)
          n73 = Unbundle By Name(w43) -> ("FreeSpeed_RadPerSec"=w75:dbl)
          n74 = Compound Arithmetic op=MULTIPLY(w64, w65) -> (w47:dbl)
          n75 = Reciprocal(x=w45) -> (1/x=w67:dbl)
          n76 = Multiply(x=w53, y=w47) -> (x*y=w52:dbl)
          n77 = Multiply(x=w54, y=w47) -> (x*y=w55:dbl)
          n78 = call <vilib>:"Units_RotationsToRadians.vi"("Rotations"=w52) -> ("Radians"=w51:dbl)  [unwired: 10 in]
          n79 = call <vilib>:"Units_RotationsToRadians.vi"("Rotations"=w55) -> ("Radians"=w63:dbl)  [unwired: 10 in]
          n80 = Compound Arithmetic op=MULTIPLY(w75, w67) -> (w74:dbl)
          n81 = Reciprocal(x=w74) -> (1/x=w72:dbl)
          n82 = Add(x=w50, y=w51) -> (x+y=w49:dbl)
          n83 = Multiply(x=1.0, y=w72) -> (x*y=w71:dbl)
          n84 = call <vilib>:"Units_RadiansToRotations.vi"("Radians"=w49) -> ("Rotations"=w48:dbl)  [unwired: 10 in]
          n85 = Divide(x=w48, y=w47) -> (x/y=w46:dbl)
          n86 = call <vilib>:"SimpleMotorFF_New.vi"("Kn"=w44, "Ka"=w76, "Kv"=w71, "Ks"=w77) -> ("SIMPLE_MOTOR_FF"=w69:T15)  [unwired: 7 in]
          n87 = call <vilib>:"SimpleMotorFF_Calculate_CalcAccel.vi"("dT_Sec"=w70, "VelSp"=w63, "SIMPLE_MOTOR_FF"=w69) -> ("FeedForward"=w68:dbl)  [unwired: 8 in]
          n88 = call <vilib>:"CTRE_Phoenix_MotorControl_RefNumRegistryGet.vi"("refnum name"=w56) -> ("error out"=w80:errorcluster, "PhoenixMotorControlDevRef"=w81:T16)  [unwired: 9 in]
          n89 = call <vilib>:"CTRE_Phoenix_MotorControl_Set.vi"("Demand1"=w68, "DemandType"=T6."DemandType_ArbitraryFeedForward", "error in (no error)"=w80, "Output"=w46, "Control Mode"=w79, "PhoenixMotorControlDevRef"=w81) -> ()  [unwired: 4 in, 2 out]
        }
        frame "Talon FX, P6" {
          w107 = 1.0  # unitless conversion
          w110 = 0.02  # dT_Sec
          w85 = 1  # Num Motors
          w117 = 0.0  # Ks
          w116 = 0.0  # Ka
          n90 = call <vilib>:"Phoenix6_Device_RefNumRegistryGet.vi"("refnum name"=w89) -> ("error out"=w92:errorcluster, "data"=w93:T21)  [unwired: 9 in]
          n91 = call-poly <vilib>:"TalonFXGetters.vi"("error in"=w92, "DeviceReference"=w93) -> ("Output"=w90:T22)  [unwired: 8 in, 1 out]
          n92 = call-poly <vilib>:"TalonFXGetters.vi"("error in"=w92, "DeviceReference"=w93) -> ("Output"=w91:T22)  [unwired: 8 in, 1 out]
          n93 = call <vilib>:"DCMotor_PickMotorSelector.vi"("DCMOTOR_TYPES"=w82, "Num Motors"=w85) -> ("DCMOTOR"=w86:T13)  [unwired: 9 in]
          n94 = Unbundle By Name(w91) -> ("Value"=w88:dbl)
          n95 = Unbundle By Name(w90) -> ()  [unwired: 1 out]
          n96 = Reciprocal(x=w107) -> (1/x=w105:dbl)
          n97 = Reciprocal(x=w95) -> (1/x=w106:dbl)
          n98 = Unbundle By Name(w86) -> ("FreeSpeed_RadPerSec"=w115:dbl)
          n99 = Compound Arithmetic op=MULTIPLY(w105, w106) -> (w96:dbl)
          n100 = Reciprocal(x=w95) -> (1/x=w108:dbl)
          n101 = Multiply(x=w88, y=w96) -> (x*y=w101:dbl)
          n102 = Multiply(x=w102, y=w96) -> (x*y=w103:dbl)
          n103 = call <vilib>:"Units_RotationsToRadians.vi"("Rotations"=w101) -> ("Radians"=w100:dbl)  [unwired: 10 in]
          n104 = call <vilib>:"Units_RotationsToRadians.vi"("Rotations"=w103) -> ("Radians"=w104:dbl)  [unwired: 10 in]
          n105 = Compound Arithmetic op=MULTIPLY(w115, w108) -> (w114:dbl)
          n106 = Reciprocal(x=w114) -> (1/x=w112:dbl)
          n107 = Add(x=w99, y=w100) -> (x+y=w98:dbl)
          n108 = Multiply(x=1.0, y=w112) -> (x*y=w111:dbl)
          n109 = call <vilib>:"Units_RadiansToRotations.vi"("Radians"=w98) -> ("Rotations"=w97:dbl)  [unwired: 10 in]
          n110 = Divide(x=w97, y=w96) -> (x/y=w84:dbl)
          n111 = call <vilib>:"SimpleMotorFF_New.vi"("Kn"=w94, "Ka"=w116, "Kv"=w111, "Ks"=w117) -> ("SIMPLE_MOTOR_FF"=w109:T15)  [unwired: 7 in]
          n112 = call <vilib>:"SimpleMotorFF_Calculate_CalcAccel.vi"("dT_Sec"=w110, "VelSp"=w104, "SIMPLE_MOTOR_FF"=w109) -> ("FeedForward"=w83:dbl)  [unwired: 8 in]
          n113 = call <vilib>:"Phoenix6_Device_RefNumRegistryGet.vi"("refnum name"=w89) -> ("data"=w87:T21)  [unwired: 9 in, 1 out]
          n114 = call-poly <vilib>:"TalonFXSetter.vi"("DeviceReference"=w87, "Position"=w84, "FeedForward"=w83) -> ()  [unwired: 23 in, 2 out]
        }
        frame "SPARK MAX" {
          w140 = 1.0  # unitless conversion
          w143 = 0.02  # dT_Sec
          w147 = 12.0  # Nominal Voltage
          w123 = 1  # Num Motors
          w151 = 0.0  # Ks
          w150 = 0.0  # Ka
          n115 = call <vilib>:"WPI_MotorControlRefNum Registry Get.vi"("refnum name"=w136) -> ("error out"=w119:errorcluster, "MotorControlDevRef"=w118:T16)  [unwired: 9 in]
          n116 = call-poly <vilib>:"SPARK Get Encoder Status.vi"("MotorControlDevRef in"=w118) -> ("Sensor Position"=w121:dbl)  [unwired: 7 in, 3 out]
          n117 = call-poly <vilib>:"SPARK Get Encoder Status.vi"("error in (no error)"=w119, "MotorControlDevRef in"=w118) -> ("Sensor Velocity"=w120:dbl)  [unwired: 6 in, 3 out]
          n118 = call <vilib>:"Units_RotationsPerMinuteToRadiansPerSecond.vi"("RotationsPerMinute"=w120) -> ()  [unwired: 10 in, 1 out]
          n119 = call <vilib>:"DCMotor_PickMotorSelector.vi"("DCMOTOR_TYPES"=w122, "Num Motors"=w123) -> ("DCMOTOR"=w124:T13)  [unwired: 9 in]
          n120 = Reciprocal(x=w140) -> (1/x=w138:dbl)
          n121 = Reciprocal(x=w126) -> (1/x=w139:dbl)
          n122 = Unbundle By Name(w124) -> ("FreeSpeed_RadPerSec"=w149:dbl)
          n123 = Compound Arithmetic op=MULTIPLY(w138, w139) -> (w128:dbl)
          n124 = Reciprocal(x=w126) -> (1/x=w144:dbl)
          n125 = Multiply(x=w121, y=w128) -> (x*y=w133:dbl)
          n126 = Multiply(x=w135, y=w128) -> (x*y=w134:dbl)
          n127 = call <vilib>:"Units_RotationsToRadians.vi"("Rotations"=w133) -> ("Radians"=w132:dbl)  [unwired: 10 in]
          n128 = call <vilib>:"Units_RotationsToRadians.vi"("Rotations"=w134) -> ("Radians"=w137:dbl)  [unwired: 10 in]
          n129 = Compound Arithmetic op=MULTIPLY(w149, w144) -> (w148:dbl)
          n130 = Reciprocal(x=w148) -> (1/x=w146:dbl)
          n131 = Add(x=w130, y=w132) -> (x+y=w131:dbl)
          n132 = Multiply(x=w147, y=w146) -> (x*y=w145:dbl)
          n133 = call <vilib>:"Units_RadiansToRotations.vi"("Radians"=w131) -> ("Rotations"=w129:dbl)  [unwired: 10 in]
          n134 = Divide(x=w129, y=w128) -> (x/y=w127:dbl)
          n135 = call <vilib>:"SimpleMotorFF_New.vi"("Kn"=w125, "Ka"=w150, "Kv"=w145, "Ks"=w151) -> ("SIMPLE_MOTOR_FF"=w142:T15)  [unwired: 7 in]
          n136 = call <vilib>:"SimpleMotorFF_Calculate_CalcAccel.vi"("dT_Sec"=w143, "VelSp"=w137, "SIMPLE_MOTOR_FF"=w142) -> ("FeedForward"=w141:dbl)  [unwired: 8 in]
          n137 = call <vilib>:"WPI_MotorControlRefNum Registry Get.vi"("refnum name"=w136) -> ("error out"=w153:errorcluster, "MotorControlDevRef"=w154:T16)  [unwired: 9 in]
          n138 = call <vilib>:"SPARK Set Output Advanced.vi"("Arbitrary Feed Forward (0)"=w141, "error in (no error)"=w153, "Control Mode"=Spark_MAX_Control_Type."Position", "Setpoint"=w127, "MotorControlDevRef"=w154) -> ()  [unwired: 5 in, 2 out]
        }
      }
    }
    frame condition #1 (active) {
      w258 = 1.0  # Kf
      w274 = 0.0  # MinInput
      w273 = FALSE  # Continuous
      w272 = 1.0  # MaxOutput
      w275 = -1.0  # MinOutput
      w271 = 0.0  # MaxInput
      w293 = 100.0  # Max Speed R/s
      w292 = 100.0  # Max Accel R/s^2
      w290 = 1.0  # MaxInput
      w289 = -1.0  # MinInput
      w288 = FALSE  # Continuous
      w302 = 12.0 ("Battery_Volts")
      w321 = 1.0  # unitless conversion
      w324 = 0.02  # dT_Sec
      w331 = 0.0  # Ks
      w330 = 0.0  # Ka
      w300 = 12.0 ("Battery_Volts")
      w345 = 0.02  # dT_Sec
      w353 = 0.01  # Ks
      w352 = 0.0  # Ka
      # "R/s"
      n139 = case shown="\"Talon FX, P5\", Default" w256 {
        tunnel: [w376 w379 w382] -> w257
        frame "Talon FX, P5", Default {
          n140 = call <vilib>:"DCMotor_PickMotorSelector.vi"("DCMOTOR_TYPES"=DCMOTOR_TYPES_ENUM."Falcon 500", "Num Motors"=1) -> ("DCMOTOR"=w376:T13)  [unwired: 9 in]
        }
        frame "Talon FX, P6" {
          n141 = call <vilib>:"DCMotor_PickMotorSelector.vi"("DCMOTOR_TYPES"=DCMOTOR_TYPES_ENUM."Kraken X60", "Num Motors"=1) -> ("DCMOTOR"=w379:T13)  [unwired: 9 in]
        }
        frame "SPARK MAX" {
          n142 = call <vilib>:"DCMotor_PickMotorSelector.vi"("DCMOTOR_TYPES"=DCMOTOR_TYPES_ENUM."NEO", "Num Motors"=1) -> ("DCMOTOR"=w382:T13)  [unwired: 9 in]
        }
      }
      n143 = case shown="\"Talon FX, P5\", Default" w254 {
        tunnel: [w367 w370 w373] -> w255
        frame "Talon FX, P5", Default {
          n144 = call <vilib>:"DCMotor_PickMotorSelector.vi"("DCMOTOR_TYPES"=DCMOTOR_TYPES_ENUM."Falcon 500", "Num Motors"=1) -> ("DCMOTOR"=w367:T13)  [unwired: 9 in]
        }
        frame "Talon FX, P6" {
          n145 = call <vilib>:"DCMotor_PickMotorSelector.vi"("DCMOTOR_TYPES"=DCMOTOR_TYPES_ENUM."Kraken X60", "Num Motors"=1) -> ("DCMOTOR"=w370:T13)  [unwired: 9 in]
        }
        frame "SPARK MAX" {
          n146 = call <vilib>:"DCMotor_PickMotorSelector.vi"("DCMOTOR_TYPES"=DCMOTOR_TYPES_ENUM."NEO", "Num Motors"=1) -> ("DCMOTOR"=w373:T13)  [unwired: 9 in]
        }
      }
      n147 = Concatenate Strings("Drive/Sim/" ("name"), w276) -> (w332:string)
      n148 = Concatenate Strings("Drive/Sim/" ("name"), w295) -> (w311:string)
      n149 = call-poly <vilib>:"NT Read Value.vi"("name"=w332) -> ("Variant"=w339:variant)  [unwired: 9 in, 1 out]
      n150 = call-poly <vilib>:"NT Read Value.vi"("name"=w311) -> ("Variant"=w304:variant)  [unwired: 9 in, 1 out]
      n151 = call <vilib>:"Units_InchesToMeters.vi"("Inches"=w362) -> ("Meters"=w356:dbl)  [unwired: 10 in]
      n152 = Variant To Data(type=T9 {"LinearSystemSim"={"m_Plant"={"m_A"=[], "m_B"=[], "m_C"=[], "m_D"=[], "States"=0, "Inputs"=0, "Outputs"=0}, "m_X"=[], "m_Y"=[], "m_U"=[], "MeasureStdDev"=[]}, "GearBox"={"nominalVoltage_Volts"=0.0, "StallTorque_NM"=0.0, "StallCurrent_Amps"=0.0, "FreeCurrent_Amps"=0.0, "FreeSpeed_RadPerSec"=0.0, "R_Ohms"=0.0, "KvINV_RadPerSecPerVolt"=0.0, "Kt_NMPerAmp"=0.0, "L_H"=0.0, "Jr_KgM2"=0.0}, "Gearing"=0.0} ("DCMOTOR_SIM"), Variant=w339) -> (data=w263:T9)  [unwired: 1 in, 1 out]
      n153 = Variant To Data(type=T9 {"LinearSystemSim"={"m_Plant"={"m_A"=[], "m_B"=[], "m_C"=[], "m_D"=[], "States"=0, "Inputs"=0, "Outputs"=0}, "m_X"=[], "m_Y"=[], "m_U"=[], "MeasureStdDev"=[]}, "GearBox"={"nominalVoltage_Volts"=0.0, "StallTorque_NM"=0.0, "StallCurrent_Amps"=0.0, "FreeCurrent_Amps"=0.0, "FreeSpeed_RadPerSec"=0.0, "R_Ohms"=0.0, "KvINV_RadPerSecPerVolt"=0.0, "Kt_NMPerAmp"=0.0, "L_H"=0.0, "Jr_KgM2"=0.0}, "Gearing"=0.0} ("DCMOTOR_SIM"), Variant=w304) -> (data=w303:T9)  [unwired: 1 in, 1 out]
      n154 = Reciprocal(x=w321) -> (1/x=w319:dbl)
      n155 = Reciprocal(x=w361) -> (1/x=w320:dbl)
      n156 = Unbundle By Name(w255) -> ("FreeSpeed_RadPerSec"=w347:dbl)
      n157 = Unbundle By Name(w257) -> ("FreeSpeed_RadPerSec"=w329:dbl)
      n158 = Divide(x=w356, y=2.0) -> (x/y=w355:dbl)
      n159 = call <vilib>:"DCMotorSim_getAngularPositionRotations.vi"("DCMotorSim"=w303) -> ("Position_Rotations"=w285:dbl)  [unwired: 10 in]
      n160 = call <vilib>:"Units_InchesToMeters.vi"("Inches"=w362) -> ("Meters"=w351:dbl)  [unwired: 10 in]
      n161 = Compound Arithmetic op=MULTIPLY(w319, w320) -> (w312:dbl)
      n162 = Reciprocal(x=w355) -> (1/x=w354:dbl)
      n163 = Divide(x=w351, y=2.0) -> (x/y=w349:dbl)
      n164 = Reciprocal(x=w360) -> (1/x=w348:dbl)
      n165 = Reciprocal(x=w361) -> (1/x=w322:dbl)
      n166 = call <vilib>:"DCMotorSim_getAngularVelocityRadPerSec.vi"("DCMotorSim"=w263) -> ("Velocity_RadPerSec"=w264:dbl)  [unwired: 10 in]
      n167 = Compound Arithmetic op=MULTIPLY(w364, w354, w360) -> (w343:dbl)
      n168 = Multiply(x=w285, y=w312) -> (x*y=w316:dbl)
      n169 = Multiply(x=w365, y=w312) -> (x*y=w317:dbl)
      n170 = Concatenate Strings("Drive/Sim/Config_" ("name"), w276) -> (w279:string)
      n171 = Concatenate Strings("Drive/Sim/Config_" ("name"), w295) -> (w296:string)
      n172 = call <vilib>:"Units_RotationsToRadians.vi"("Rotations"=w316) -> ("Radians"=w315:dbl)  [unwired: 10 in]
      n173 = call <vilib>:"Units_RotationsToRadians.vi"("Rotations"=w317) -> ("Radians"=w318:dbl)  [unwired: 10 in]
      n174 = Compound Arithmetic op=MULTIPLY(w329, w322) -> (w328:dbl)
      n175 = Compound Arithmetic op=MULTIPLY(w347, w349, w348) -> (w346:dbl)
      n176 = call <vilib>:"Units_RadiansToRotations.vi"("Radians"=w264) -> ("Rotations"=w262:dbl)  [unwired: 10 in]
      n177 = call <vilib>:"Units_RadiansToRotations.vi"("Radians"=w343) -> ("Rotations"=w261:dbl)  [unwired: 10 in]
      n178 = Reciprocal(x=w328) -> (1/x=w326:dbl)
      n179 = Reciprocal(x=w346) -> (1/x=w341:dbl)
      n180 = call-poly <vilib>:"NT Read Value.vi"("name"=w279) -> ("Variant"=w278:variant)  [unwired: 9 in, 1 out]
      n181 = call-poly <vilib>:"NT Read Value.vi"("name"=w296) -> ("Variant"=w297:variant)  [unwired: 9 in, 1 out]
      n182 = Add(x=w363, y=w315) -> (x+y=w314:dbl)
      n183 = Multiply(x=1.0, y=w326) -> (x*y=w325:dbl)
      n184 = Multiply(x=1.0, y=w341) -> (x*y=w340:dbl)
      n185 = Variant To Data(type=T8 {"Future Proof Configs"=FALSE, "MotorOutputInverted"=0, "MotorOutputNeutralMode"=0, "MotorOutputDutyCycleNeutralDeadband"=0.0, "MotorOutputPeakForwardDutyCycle"=1.0, "MotorOutputPeakReverseDutyCycle"=-1.0, "MotorOutputControlTimesyncFreqHz"=0.0, "CurrentLimitsStatorCurrentLimit"=120.0, "CurrentLimitsStatorCurrentLimitEnable"=TRUE, "CurrentLimitsSupplyCurrentLimit"=70.0, "CurrentLimitsSupplyCurrentLimitEnable"=TRUE, "CurrentLimitsSupplyCurrentLowerLimit"=40.0, "CurrentLimitsSupplyCurrentLowerTime"=1.0, "VoltageSupplyVoltageTimeConstant"=0.0, "VoltagePeakForwardVoltage"=16.0, "VoltagePeakReverseVoltage"=-16.0, "TorqueCurrentPeakForwardTorqueCurrent"=800.0, "TorqueCurrentPeakReverseTorqueCurrent"=-800.0, "TorqueCurrentTorqueNeutralDeadband"=0.0, "FeedbackFeedbackRotorOffset"=0.0, "FeedbackSensorToMechanismRatio"=1.0, "FeedbackRotorToSensorRatio"=1.0, "FeedbackFeedbackSensorSource"=0, "FeedbackFeedbackRemoteSensorID"=0, "FeedbackVelocityFilterTimeConstant"=0.0, "DifferentialSensorsDifferentialSensorSource"=0, "DifferentialSensorsDifferentialTalonFXSensorID"=0, "DifferentialSensorsDifferentialRemoteSensorID"=0, "DifferentialConstantsPeakDifferentialDutyCycle"=2.0, "DifferentialConstantsPeakDifferentialVoltage"=32.0, "DifferentialConstantsPeakDifferentialTorqueCurrent"=1600.0, "OpenLoopRampsDutyCycleOpenLoopRampPeriod"=0.0, "OpenLoopRampsVoltageOpenLoopRampPeriod"=0.0, "OpenLoopRampsTorqueOpenLoopRampPeriod"=0.0, "ClosedLoopRampsDutyCycleClosedLoopRampPeriod"=0.0, "ClosedLoopRampsVoltageClosedLoopRampPeriod"=0.0, "ClosedLoopRampsTorqueClosedLoopRampPeriod"=0.0, "HardwareLimitSwitchForwardLimitType"=0, "HardwareLimitSwitchForwardLimitAutosetPositionEnable"=FALSE, "HardwareLimitSwitchForwardLimitAutosetPositionValue"=0.0, "HardwareLimitSwitchForwardLimitEnable"=TRUE, "HardwareLimitSwitchForwardLimitSource"=0, "HardwareLimitSwitchForwardLimitRemoteSensorID"=0, "HardwareLimitSwitchReverseLimitType"=0, "HardwareLimitSwitchReverseLimitAutosetPositionEnable"=FALSE, "HardwareLimitSwitchReverseLimitAutosetPositionValue"=0.0, "HardwareLimitSwitchReverseLimitEnable"=TRUE, "HardwareLimitSwitchReverseLimitSource"=0, "HardwareLimitSwitchReverseLimitRemoteSensorID"=0, "AudioBeepOnBoot"=TRUE, "AudioBeepOnConfig"=TRUE, "AudioAllowMusicDurDisable"=FALSE, "SoftwareLimitSwitchForwardSoftLimitEnable"=FALSE, "SoftwareLimitSwitchReverseSoftLimitEnable"=FALSE, "SoftwareLimitSwitchForwardSoftLimitThreshold"=0.0, "SoftwareLimitSwitchReverseSoftLimitThreshold"=0.0, "MotionMagicMotionMagicCruiseVelocity"=0.0, "MotionMagicMotionMagicAcceleration"=0.0, "MotionMagicMotionMagicJerk"=0.0, "MotionMagicMotionMagicExpo_kV"=0.12, "MotionMagicMotionMagicExpo_kA"=0.1, "CustomParamsCustomParam0"=0, "CustomParamsCustomParam1"=0, "ClosedLoopGeneralContinuousWrap"=FALSE, "Slot0kP"=0.0, "Slot0kI"=0.0, "Slot0kD"=0.0, "Slot0kS"=0.0, "Slot0kV"=0.0, "Slot0kA"=0.0, "Slot0kG"=0.0, "Slot0GravityType"=0, "Slot0StaticFeedforwardSign"=0, "Slot1kP"=0.0, "Slot1kI"=0.0, "Slot1kD"=0.0, "Slot1kS"=0.0, "Slot1kV"=0.0, "Slot1kA"=0.0, "Slot1kG"=0.0, "Slot1GravityType"=0, "Slot1StaticFeedforwardSign"=0, "Slot2kP"=0.0, "Slot2kI"=0.0, "Slot2kD"=0.0, "Slot2kS"=0.0, "Slot2kV"=0.0, "Slot2kA"=0.0, "Slot2kG"=0.0, "Slot2GravityType"=0, "Slot2StaticFeedforwardSign"=0} ("DeviceConfiguration"), Variant=w278) -> (data=w280:T8)  [unwired: 1 in, 1 out]
      n186 = Variant To Data(type=T8 {"Future Proof Configs"=FALSE, "MotorOutputInverted"=0, "MotorOutputNeutralMode"=0, "MotorOutputDutyCycleNeutralDeadband"=0.0, "MotorOutputPeakForwardDutyCycle"=1.0, "MotorOutputPeakReverseDutyCycle"=-1.0, "MotorOutputControlTimesyncFreqHz"=0.0, "CurrentLimitsStatorCurrentLimit"=120.0, "CurrentLimitsStatorCurrentLimitEnable"=TRUE, "CurrentLimitsSupplyCurrentLimit"=70.0, "CurrentLimitsSupplyCurrentLimitEnable"=TRUE, "CurrentLimitsSupplyCurrentLowerLimit"=40.0, "CurrentLimitsSupplyCurrentLowerTime"=1.0, "VoltageSupplyVoltageTimeConstant"=0.0, "VoltagePeakForwardVoltage"=16.0, "VoltagePeakReverseVoltage"=-16.0, "TorqueCurrentPeakForwardTorqueCurrent"=800.0, "TorqueCurrentPeakReverseTorqueCurrent"=-800.0, "TorqueCurrentTorqueNeutralDeadband"=0.0, "FeedbackFeedbackRotorOffset"=0.0, "FeedbackSensorToMechanismRatio"=1.0, "FeedbackRotorToSensorRatio"=1.0, "FeedbackFeedbackSensorSource"=0, "FeedbackFeedbackRemoteSensorID"=0, "FeedbackVelocityFilterTimeConstant"=0.0, "DifferentialSensorsDifferentialSensorSource"=0, "DifferentialSensorsDifferentialTalonFXSensorID"=0, "DifferentialSensorsDifferentialRemoteSensorID"=0, "DifferentialConstantsPeakDifferentialDutyCycle"=2.0, "DifferentialConstantsPeakDifferentialVoltage"=32.0, "DifferentialConstantsPeakDifferentialTorqueCurrent"=1600.0, "OpenLoopRampsDutyCycleOpenLoopRampPeriod"=0.0, "OpenLoopRampsVoltageOpenLoopRampPeriod"=0.0, "OpenLoopRampsTorqueOpenLoopRampPeriod"=0.0, "ClosedLoopRampsDutyCycleClosedLoopRampPeriod"=0.0, "ClosedLoopRampsVoltageClosedLoopRampPeriod"=0.0, "ClosedLoopRampsTorqueClosedLoopRampPeriod"=0.0, "HardwareLimitSwitchForwardLimitType"=0, "HardwareLimitSwitchForwardLimitAutosetPositionEnable"=FALSE, "HardwareLimitSwitchForwardLimitAutosetPositionValue"=0.0, "HardwareLimitSwitchForwardLimitEnable"=TRUE, "HardwareLimitSwitchForwardLimitSource"=0, "HardwareLimitSwitchForwardLimitRemoteSensorID"=0, "HardwareLimitSwitchReverseLimitType"=0, "HardwareLimitSwitchReverseLimitAutosetPositionEnable"=FALSE, "HardwareLimitSwitchReverseLimitAutosetPositionValue"=0.0, "HardwareLimitSwitchReverseLimitEnable"=TRUE, "HardwareLimitSwitchReverseLimitSource"=0, "HardwareLimitSwitchReverseLimitRemoteSensorID"=0, "AudioBeepOnBoot"=TRUE, "AudioBeepOnConfig"=TRUE, "AudioAllowMusicDurDisable"=FALSE, "SoftwareLimitSwitchForwardSoftLimitEnable"=FALSE, "SoftwareLimitSwitchReverseSoftLimitEnable"=FALSE, "SoftwareLimitSwitchForwardSoftLimitThreshold"=0.0, "SoftwareLimitSwitchReverseSoftLimitThreshold"=0.0, "MotionMagicMotionMagicCruiseVelocity"=0.0, "MotionMagicMotionMagicAcceleration"=0.0, "MotionMagicMotionMagicJerk"=0.0, "MotionMagicMotionMagicExpo_kV"=0.12, "MotionMagicMotionMagicExpo_kA"=0.1, "CustomParamsCustomParam0"=0, "CustomParamsCustomParam1"=0, "ClosedLoopGeneralContinuousWrap"=FALSE, "Slot0kP"=0.0, "Slot0kI"=0.0, "Slot0kD"=0.0, "Slot0kS"=0.0, "Slot0kV"=0.0, "Slot0kA"=0.0, "Slot0kG"=0.0, "Slot0GravityType"=0, "Slot0StaticFeedforwardSign"=0, "Slot1kP"=0.0, "Slot1kI"=0.0, "Slot1kD"=0.0, "Slot1kS"=0.0, "Slot1kV"=0.0, "Slot1kA"=0.0, "Slot1kG"=0.0, "Slot1GravityType"=0, "Slot1StaticFeedforwardSign"=0, "Slot2kP"=0.0, "Slot2kI"=0.0, "Slot2kD"=0.0, "Slot2kS"=0.0, "Slot2kV"=0.0, "Slot2kA"=0.0, "Slot2kG"=0.0, "Slot2GravityType"=0, "Slot2StaticFeedforwardSign"=0} ("DeviceConfiguration"), Variant=w297) -> (data=w294:T8)  [unwired: 1 in, 1 out]
      n187 = call <vilib>:"Units_RadiansToRotations.vi"("Radians"=w314) -> ("Rotations"=w313:dbl)  [unwired: 10 in]
      n188 = Unbundle By Name(w280) -> ("Slot0kP"=w268:dbl, "Slot0kI"=w267:dbl, "Slot0kD"=w266:dbl)
      n189 = Unbundle By Name(w294) -> ("Slot0kP"=w283:dbl, "Slot0kI"=w282:dbl, "Slot0kD"=w281:dbl)
      n190 = Divide(x=w313, y=w312) -> (x/y=w265:dbl)
      n191 = call <vilib>:"SimpleMotorFF_New.vi"("Kn"=w359, "Ka"=w330, "Kv"=w325, "Ks"=w331) -> ("SIMPLE_MOTOR_FF"=w323:T15)  [unwired: 7 in]
      n192 = call <vilib>:"SimpleMotorFF_New.vi"("Kn"=w358, "Ka"=w352, "Kv"=w340, "Ks"=w353) -> ("SIMPLE_MOTOR_FF"=w344:T15)  [unwired: 7 in]
      n193 = call <vilib>:"SimpleMotorFF_Calculate_CalcAccel.vi"("dT_Sec"=w324, "VelSp"=w318, "SIMPLE_MOTOR_FF"=w323) -> ()  [unwired: 8 in, 1 out]
      n194 = call <vilib>:"PIDController_Pack_AdvTuning.vi"("Kf"=w258, "Kd"=w266, "Ki"=w267, "Kp"=w268) -> ("Adv PID Tuning"=w270:T23)  [unwired: 7 in]
      n195 = call <vilib>:"SimpleMotorFF_Calculate_CalcAccel.vi"("dT_Sec"=w345, "VelSp"=w364, "SIMPLE_MOTOR_FF"=w344) -> ("FeedForward"=w260:dbl)  [unwired: 8 in]
      n196 = call <vilib>:"TrapProfConstraint_New.vi"("Max Accel"=w292, "Max Speed (M/S)"=w293) -> ("TRAPEZOID_PROFILE_CONSTRAINT"=w291:T24)  [unwired: 9 in]
      n197 = call <vilib>:"PIDController_Pack_InputLimits.vi"("Continuous"=w288, "MinInput"=w289, "MaxInput"=w290) -> ("PID Input Limits"=w286:T25)  [unwired: 8 in]
      n198 = call <vilib>:"PIDController_Pack_Tuning.vi"("Kd"=w281, "Ki"=w282, "Kp"=w283) -> ("PID Tuning"=w287:T26)  [unwired: 8 in]
      n199 = call <vilib>:"PIDController_Pack_AdvLimits.vi"("MinOutput"=w275, "MaxOutput"=w272, "Continuous"=w273, "MinInput"=w274, "MaxInput"=w271) -> ("Adv PID Limits"=w269:T27)  [unwired: 6 in]
      n200 = call <vilib>:"PIDController_AdvExecute.vi"("Adv PID Limits"=w269, "FF-FeedForward"=w260, "SP-SetPoint"=w261, "PV-Measurement"=w262, "Adv PID Tuning"=w270) -> ("CO-ControlOutput"=w259:dbl)  [unwired: 4 in, 2 out]
      n201 = call <vilib>:"ProfiledPIDController_Execute.vi"("Constraints"=w291, "PID Input Limits"=w286, "SP-SetPoint Goal"=w265, "PV-Measurement"=w285, "PID Tuning"=w287) -> ("CO-ControlOutput"=w284:dbl)  [unwired: 3 in, 3 out]
      n202 = Multiply(x=w259, y=w300) -> (x*y=w299:dbl)
      n203 = Multiply(x=w284, y=w302) -> (x*y=w301:dbl)
      n204 = call <vilib>:"DCMotorSim_SetInputVoltage.vi"("Battery_Volts"=w300, "Volts"=w299, "DCMotorSim"=w263) -> ("out DCMotorSim"=w336:T9)  [unwired: 8 in]
      n205 = call <vilib>:"DCMotorSim_SetInputVoltage.vi"("Battery_Volts"=w302, "Volts"=w301, "DCMotorSim"=w303) -> ("out DCMotorSim"=w307:T9)  [unwired: 8 in]
      n206 = call <vilib>:"DCMotorSim_Update.vi"("dT_Seconds"=0.02, "DCMotorSim"=w336) -> ("out DCMotorSim"=w333:T9)  [unwired: 8 in, 1 out]
      n207 = call <vilib>:"DCMotorSim_Update.vi"("dT_Seconds"=0.02, "DCMotorSim"=w307) -> ("out DCMotorSim"=w310:T9)  [unwired: 8 in, 1 out]
      n208 = To Variant(anything=w333) -> (Variant=w334:variant)
      n209 = To Variant(anything=w310) -> (Variant=w309:variant)
      n210 = call-poly <vilib>:"NT Write Value.vi"("variant"=w334, "name"=w332) -> ()  [unwired: 9 in, 1 out]
      n211 = call-poly <vilib>:"NT Write Value.vi"("variant"=w309, "name"=w311) -> ()  [unwired: 9 in, 1 out]
    }
  }
